vi "lowpas.vi"(1 "alpha":dbl=0.9, 2 "x":dbl) -> (6 "Numeric":dbl)   [LabVIEW 2020]
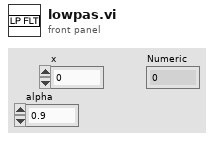
[diagram p1: front panel]
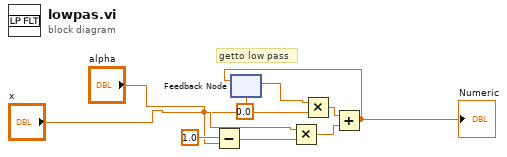
[diagram p0: block diagram]
diagram:
  # "getto low pass"
  n1 = Subtract(x=1.0, y="alpha") -> (x-y=w8:dbl)
  n2 = feedback #1(0.0) -> (w2:dbl)
  n3 = Multiply(x="x", y=w8) -> (x*y=w4:dbl)
  n4 = Multiply(x=w2, y="alpha") -> (x*y=w3:dbl)
  n5 = Add(x=w3, y=w4) -> (x+y=w6:dbl)
  "Numeric" <- w6
  n6 = feedback-in #1(w6) -> ()
